vi "AO_StreamingBufferedWrite.vi"(8 "error in (no error)":errorcluster, 9 "stop?":bool, 10 "data in(DDT)":dynamicdata(waveform), 11 "Task ID":u32) -> (0 "error out":errorcluster, 2 "stopped":bool, 3 "Task out ID":u32)   [LabVIEW 2015]
panel:
  out "status":bool
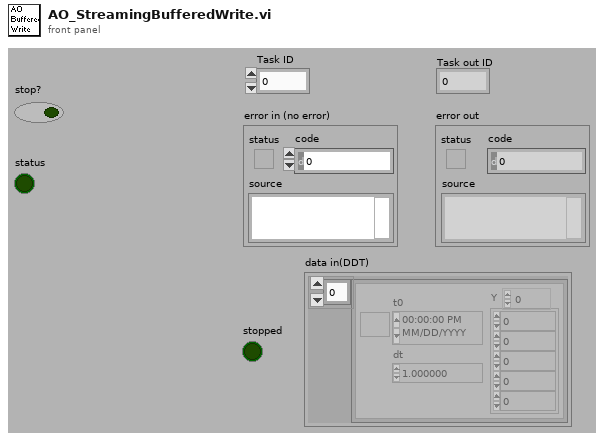
[diagram p1: front panel]
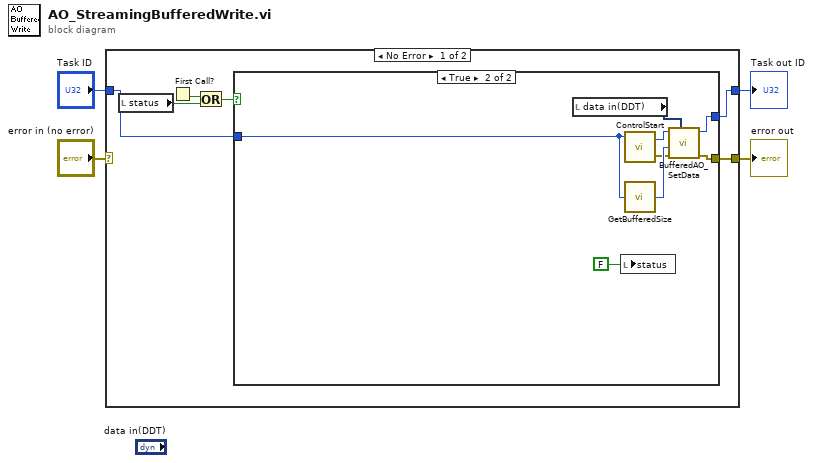
[diagram p0: block diagram]
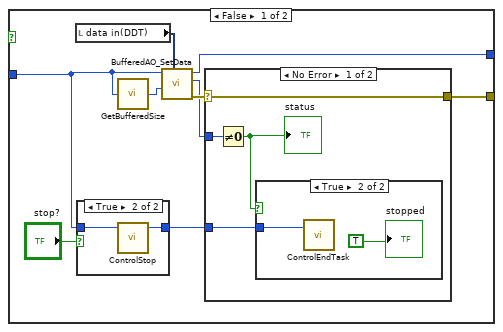
[diagram p2: hidden frame]
diagram:
  n1 = case shown="No Error" "error in (no error)" {
    selector: "error in (no error)" -> [_ w38]
    tunnel: "Task ID" -> [w10 w39]
    tunnel: [w8 w39] -> w2
    tunnel: [w9 w38] -> w1
    frame No Error {
      n2 = local read "status"() -> (w5:bool)
      n3 = First Call?() -> (First Call?: T/F=w7:bool)
      n4 = Or(x=w7, y=w5) -> (x .or. y?=w6:bool)
      n5 = case shown="True" w6 {
        tunnel: w10 -> [w18 w35]
        tunnel: [w16 w32] -> w8
        tunnel: [w13 w31] -> w9
        frame False {
          n6 = local read "data in(DDT)"() -> (w17:dynamicdata)
          n7 = case shown="True" "stop?" {
            tunnel: [w27 w29] -> w14
            tunnel: w18 -> [w27 w28]
            frame False {
            }
            frame True {
              n8 = call "ControlStop.vi"("Task ID"=w28) -> ("Task ID"=w29:u32)  [unwired: 1 in, 3 out]
            }
          }
          n9 = call "GetBufferedSize.vi"("Task ID"=w18) -> ("return type"=w11:i32)
          n10 = call "BufferedAO_SetData.vi"("data in(DDT)"=w17, "count"=w11, "Task ID"=w18) -> ("error out"=w15:errorcluster, "remaining count"=w12:i32, "Task ID"=w16:u32)  [unwired: 2 in, 4 out]
          n11 = case shown="No Error" w15 {
            selector: w15 -> [w21 w26]
            tunnel: w14 -> [w23 _]
            tunnel: [w21 w26] -> w13
            tunnel: w12 -> [w22 _]
            frame No Error {
              n12 = Not Equal To 0?(x=w22) -> (x != 0?=w20:bool)
              "status" <- w20
              n13 = case shown="True" w20 {
                tunnel: w23 -> [_ w25]
                frame False {
                }
                frame True {
                  n14 = call "ControlEndTask.vi"("Task ID"=w25) -> ()  [unwired: 1 in, 2 out]
                  "stopped" <- TRUE ("stopped")
                }
              }
            }
            frame Error {
            }
          }
        }
        frame True {
          n15 = local read "data in(DDT)"() -> (w36:dynamicdata)
          n16 = local write "status"(FALSE ("status")) -> ()
          n17 = call "ControlStart.vi"("Task ID"=w35) -> ("error out"=w33:errorcluster, "Task ID"=w34:u32)  [unwired: 1 in, 1 out]
          n18 = call "GetBufferedSize.vi"("Task ID"=w35) -> ("return type"=w37:i32)
          n19 = call "BufferedAO_SetData.vi"("data in(DDT)"=w36, "error in (no error)"=w33, "count"=w37, "Task ID"=w34) -> ("error out"=w31:errorcluster, "Task ID"=w32:u32)  [unwired: 1 in, 5 out]
        }
      }
    }
    frame Error {
    }
  }
  "Task out ID" <- w2
  "error out" <- w1
